vi "Configure Voltage Measurement (Average).vi"(7 "Enable Moving Average Filter (F: Disable)":bool, 8 "error in (no error)":errorcluster, 9 "Moving Average Count (1)":i32=1, 10 "Channel (1: Channel 1)":i32(ring)=1 items=["Channel 1"=1, "Channel 2"=2], 11 "VISA resource name":refnum<visa-resource-name>) -> (0 "error out":errorcluster, 3 "VISA resource name out":refnum<visa-resource-name>)   [LabVIEW 2012, in "Keysight B2980 Series.lvlib"]
doc: "Configures the average settings for voltage measurement function.\n\n<b>Note(s):</b>\n(1) This VI is only applicable for model B2985A and B2987A.\n(2) Voltage measurement should be enabled from <b>Configure Measurement Function.vi</b>."
uses:
  Keysight B2980 Series.lvlib
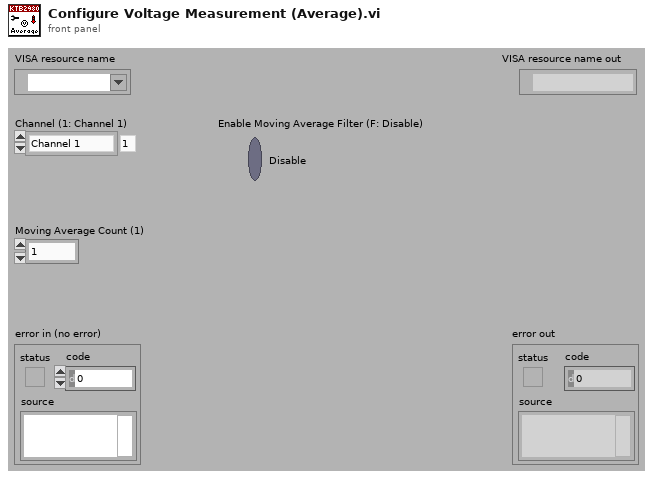
[diagram p1: front panel]
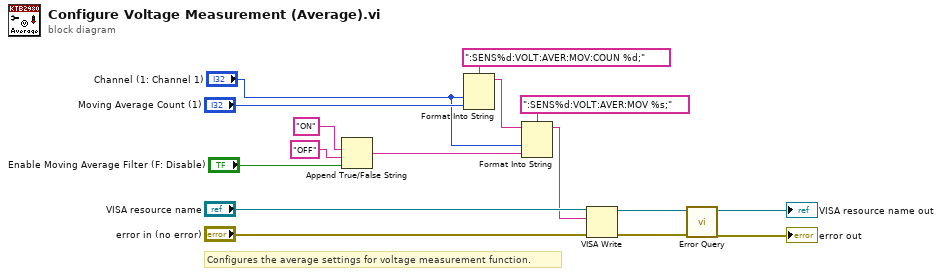
[diagram p0: block diagram]
diagram:
  # "Configures the average settings for voltage measurement function."
  n1 = Append True/False String(1:"Enable Moving Average Filter (F: Disable)", 2:"OFF", 3:"ON") -> (0:w5:string)  [unwired: 1 out]
  n2 = Format Into String(format string=":SENS%d:VOLT:AVER:MOV:COUN %d;", "Channel (1: Channel 1)", "Moving Average Count (1)") -> (resulting string=w7:string)  [unwired: 2 in, 1 out]
  n3 = Format Into String(format string=":SENS%d:VOLT:AVER:MOV %s;", initial string=w7, "Channel (1: Channel 1)", w5) -> (resulting string=w1:string)  [unwired: 1 in, 1 out]
  n4 = VISA Write(VISA resource name="VISA resource name", write buffer=w1, error in (no error)="error in (no error)") -> (VISA resource name out=w14:refnum<visa-resource-name>, error out=w13:errorcluster)  [unwired: 1 out]
  n5 = call "Error Query.vi"("error in (no error)"=w13, "VISA resource name"=w14) -> ("error out"=→"error out":errorcluster, "VISA resource name out"=→"VISA resource name out":refnum<visa-resource-name>)  [unwired: 8 out]
